vi "Receive (TDM).vi"(6 "ready for output":bool, 7 "configuration":T1={"number of channels"=2, "bits per channel"=16, "data sample edge"=enum."rising", "frame start delay"=0, "inverted sync"=FALSE}, 9 "receive":bool, 11 "signals in":cluster{"clock":bool, "sync":bool, "sdata":bool}) -> (1 "output valid":bool, 3 "sample":u32)   [LabVIEW 2013, in "I2S-TDM.lvlib"]
uses:
  I2S-TDM.lvlib
  Controls/receiver configuration.ctl
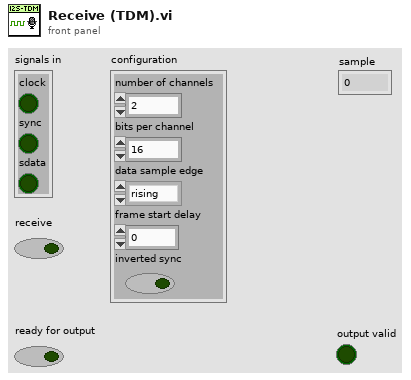
[diagram p1: front panel]
types:
  T1 = typedef "I2S-TDM.lvlib/receiver configuration.ctl" = cluster{"number of channels":u8, "bits per channel":u8, "data sample edge":enum16{"rising", "falling"}, "frame start delay":u8, "inverted sync":bool}
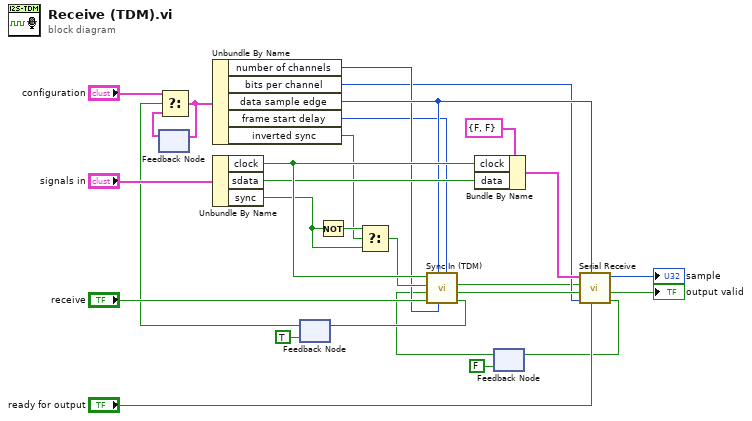
[diagram p0: block diagram]
diagram:
  n1 = feedback #1() -> (w10:T1)  [unwired: 1 in]
  n2 = Unbundle By Name("signals in") -> ("clock"=w25:bool, "sdata"=w24:bool, "sync"=w18:bool)
  n3 = feedback #2(TRUE ("latch config")) -> (w9:bool)
  n4 = Select(t="configuration", s=w9, f=w10) -> (s? t:f=w11:T1)
  n5 = feedback-in #1(w11) -> ()
  n6 = Unbundle By Name(w11) -> ("number of channels"=w19:u8, "bits per channel"=w14:u8, "data sample edge"=w22:enum16{"rising", "falling"}, "frame start delay"=w5:u8, "inverted sync"=w16:bool)
  n7 = Not(x=w18) -> (.not. x?=w17:bool)
  n8 = Select(t=w17, s=w16, f=w18) -> (s? t:f=w20:bool)
  n9 = Bundle By Name(cluster=cluster{"clock":bool, "data":bool} {"clock"=FALSE, "data"=FALSE} ("signals in"), "clock"=w25, "data"=w24) -> (w23:cluster{"clock":bool, "data":bool})
  n10 = feedback #3(FALSE ("latch config")) -> (w7:bool)
  n11 = call "Sync In (TDM).vi"("start delay (0)"=w5, "channel count (2)"=w19, "data sample edge (rising)"=w22, "receive"="receive", "prev transfer done"=w7, "frame sync in"=w20, "clock in"=w25) -> ("latch config"=w13:bool, "force output"=w15:bool, "start read"=w1:bool)  [unwired: 2 in]
  n12 = feedback-in #2(w13) -> ()
  n13 = call "Serial Receive.vi"("ready for output"="ready for output", "data sampling edge"=w22, "transfer length"=w14, "force stop (F)"=w15, "start transfer"=w1, "signals in"=w23) -> ("transfer done"=w3:bool, "output valid"=→"output valid":bool, "sample out"=→"sample":u32)  [unwired: 3 in]
  n14 = feedback-in #3(w3) -> ()
